vi "ProgressBar.vi"(2 "Time_end":dbl, 3 "TimeBegin":u32) -> (0 "TrueFalse":bool, 1 "Stabilisation Bar":u8)   [LabVIEW 2018]
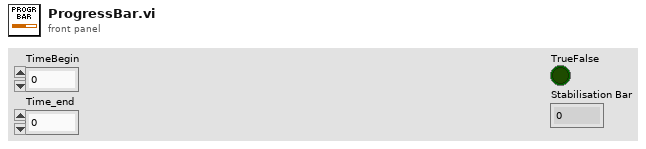
[diagram p1: front panel]
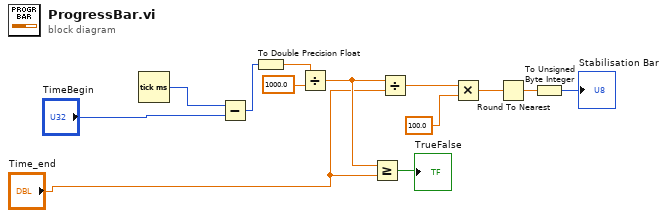
[diagram p0: block diagram]
diagram:
  n1 = Tick Count (ms)() -> (millisecond timer value=w13:u32)
  n2 = Subtract(x=w13, y="TimeBegin") -> (x-y=w7:u32)
  n3 = To Double Precision Float(number=w7) -> (double precision float=w8:dbl)
  n4 = Divide(x=w8, y=1000.0) -> (x/y=w5:dbl)
  n5 = Greater Or Equal?(x=w5, y="Time_end") -> (x >= y?=→"TrueFalse":bool)
  n6 = Divide(x=w5, y="Time_end") -> (x/y=w11:dbl)
  n7 = Multiply(x=w11, y=100.0) -> (x*y=w10:dbl)
  n8 = Round To Nearest(number=w10) -> (nearest integer value=w9:dbl)
  n9 = To Unsigned Byte Integer(number=w9) -> (unsigned 8bit integer=→"Stabilisation Bar":u8)
